vi "lavaggiolezzovi.vi"() -> ()   [LabVIEW 2012]
panel:
  in  "Slide":dbl(slide) scale=0.0..100.0
  in  "stop":bool
  out "Stato":string
  in  "Avvia Acqua sapone e spazzole":bool
  in  "Avanza auto":bool
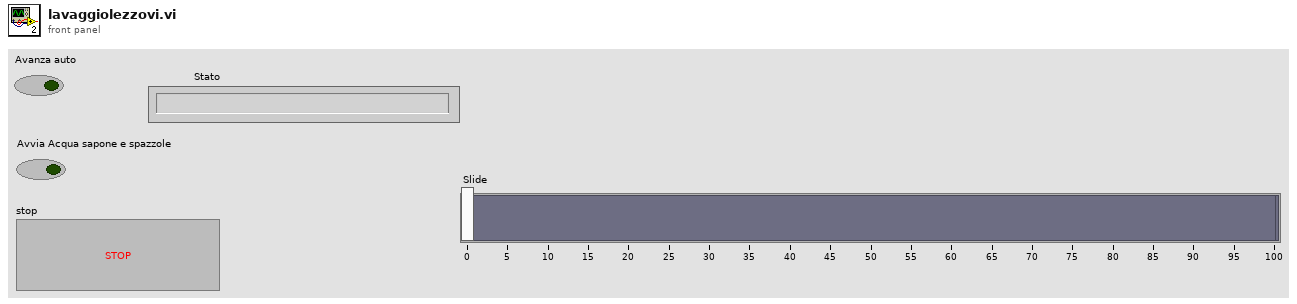
[diagram p1: front panel]
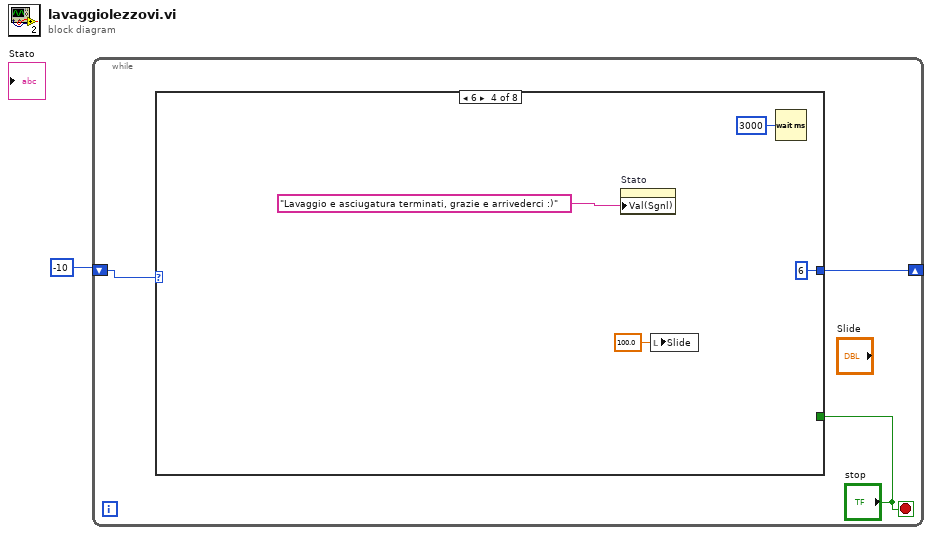
[diagram p0: block diagram]
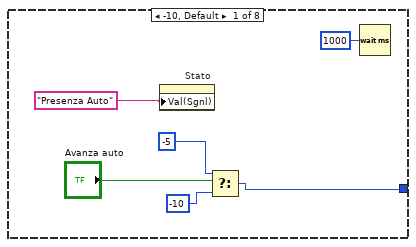
[diagram p2: hidden frame]
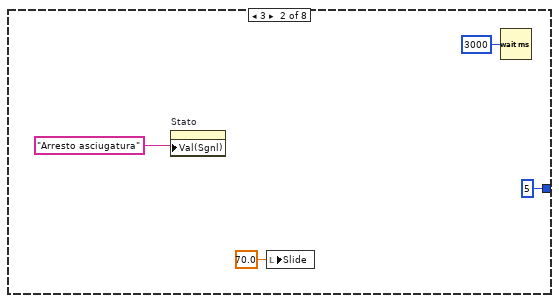
[diagram p3: hidden frame]
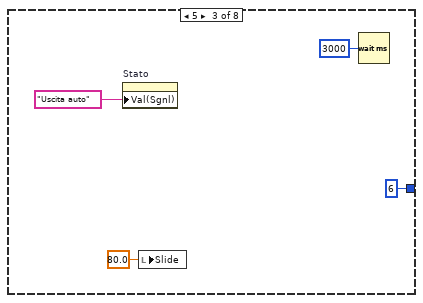
[diagram p4: hidden frame]
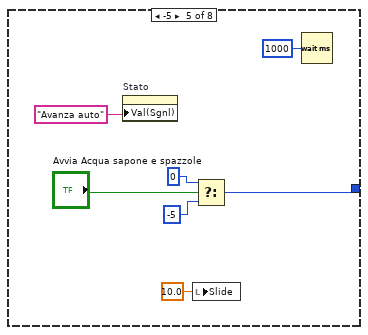
[diagram p5: hidden frame]
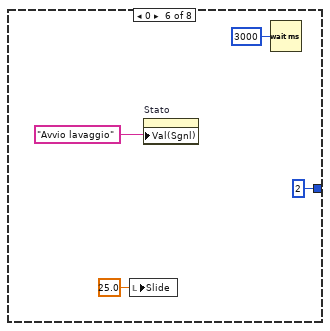
[diagram p6: hidden frame]
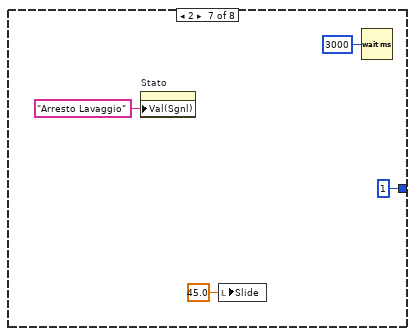
[diagram p7: hidden frame]
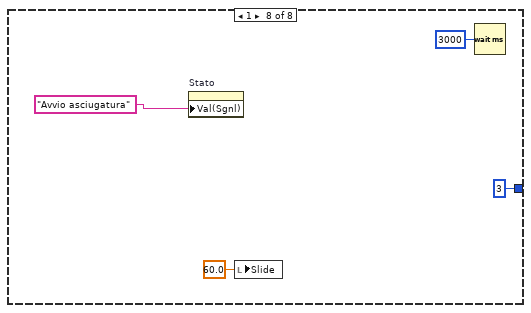
[diagram p8: hidden frame]
diagram:
  n1 = while {
    shift-right: [w3] -> _
    shift-left: -10 -> [w4]
    stop <- "stop" stop-if-true
    n2 = case shown="6" w4 {
      tunnel: [w8 5 6 6 ("t") w26 2 1 ("t") 3] -> w3
      tunnel: "stop" -> [_ _ _ _ _ _ _ _]
      frame -10, Default {
        n3 = property on="Stato" class="Str"("Val(Sgnl)"="Presenza Auto" ("Stato")) -> ()  [unwired: 2 in, 2 out]
        n4 = Select(t=-5, s="Avanza auto", f=-10) -> (s? t:f=w8:i32)
        n5 = Wait (ms)(milliseconds to wait=u32 1000) -> ()  [unwired: 1 out]
      }
      frame 3 {
        n6 = property on="Stato" class="Str"("Val(Sgnl)"="Arresto asciugatura" ("Stato")) -> ()  [unwired: 2 in, 2 out]
        n7 = local write "Slide"(70.0 ("Slide")) -> ()
        n8 = Wait (ms)(milliseconds to wait=u32 3000) -> ()  [unwired: 1 out]
      }
      frame 5 {
        n9 = property on="Stato" class="Str"("Val(Sgnl)"="Uscita auto" ("Stato")) -> ()  [unwired: 2 in, 2 out]
        n10 = local write "Slide"(80.0 ("Slide")) -> ()
        n11 = Wait (ms)(milliseconds to wait=u32 3000) -> ()  [unwired: 1 out]
      }
      frame 6 {
        n12 = property on="Stato" class="Str"("Val(Sgnl)"="Lavaggio e asciugatura terminati, grazie e arrivederci :)" ("Value (Signaling)")) -> ()  [unwired: 2 in, 2 out]
        n13 = local write "Slide"(100.0 ("Slide")) -> ()
        n14 = Wait (ms)(milliseconds to wait=u32 3000) -> ()  [unwired: 1 out]
      }
      frame -5 {
        n15 = property on="Stato" class="Str"("Val(Sgnl)"="Avanza auto" ("Stato")) -> ()  [unwired: 2 in, 2 out]
        n16 = local write "Slide"(10.0 ("Slide")) -> ()
        n17 = Select(t=0, s="Avvia Acqua sapone e spazzole", f=-5) -> (s? t:f=w26:i32)
        n18 = Wait (ms)(milliseconds to wait=u32 1000) -> ()  [unwired: 1 out]
      }
      frame 0 {
        n19 = local write "Slide"(25.0 ("Slide")) -> ()
        n20 = property on="Stato" class="Str"("Val(Sgnl)"="Avvio lavaggio") -> ()  [unwired: 2 in, 2 out]
        n21 = Wait (ms)(milliseconds to wait=u32 3000) -> ()  [unwired: 1 out]
      }
      frame 2 {
        n22 = property on="Stato" class="Str"("Val(Sgnl)"="Arresto Lavaggio" ("Value (Signaling)")) -> ()  [unwired: 2 in, 2 out]
        n23 = local write "Slide"(45.0 ("Slide")) -> ()
        n24 = Wait (ms)(milliseconds to wait=u32 3000) -> ()  [unwired: 1 out]
      }
      frame 1 {
        n25 = property on="Stato" class="Str"("Val(Sgnl)"="Avvio asciugatura" ("Stato")) -> ()  [unwired: 2 in, 2 out]
        n26 = local write "Slide"(60.0 ("Slide")) -> ()
        n27 = Wait (ms)(milliseconds to wait=u32 3000) -> ()  [unwired: 1 out]
      }
    }
  }
